vi "commit settings.vi"(8 "error in (no error)":errorcluster, 11 "Builders in":refnum<class "Builder.lvclass">) -> (0 "error out":errorcluster, 2 "Destinations":T1[](array[typedef]), 3 "Builders out":refnum<class "Builder.lvclass">)   [LabVIEW 2024, in "Builder.lvclass"]
uses:
  Builder.lvclass
  Builder.lvclass/Builder.ctl
  <vilib>/AppBuilder/AB_API/common/AB_API Destination Type.ctl
  <vilib>/AppBuilder/AB_API/common/AB_API Destination Data.ctl
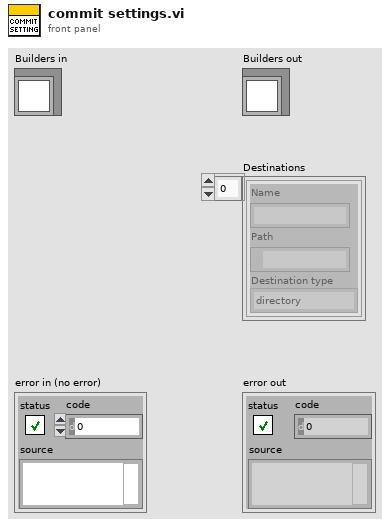
[diagram p1: front panel]
types:
  T1 = typedef "AB_API Destination Data.ctl" = cluster{"Name":string, "Path":path, "Destination type":T2}
  T2 = typedef "AB_API Destination Type.ctl" = enum16{"directory", "directory (preserve hierarchy)", "LLB"}
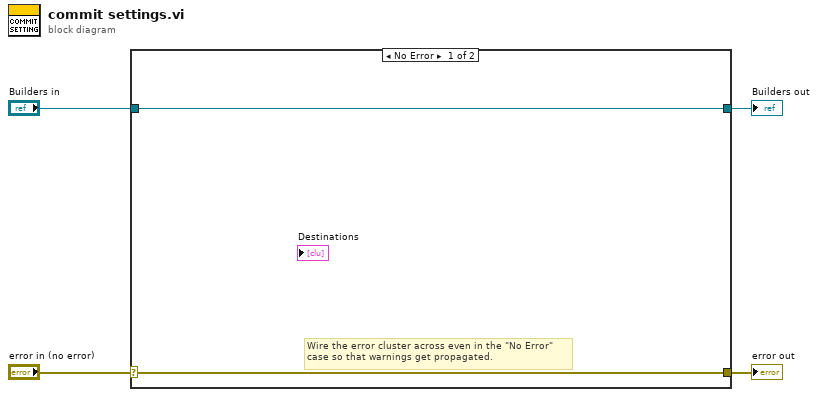
[diagram p0: block diagram]
diagram:
  n1 = case shown="No Error" "error in (no error)" {
    selector: "error in (no error)" -> [w5 w8]
    tunnel: [w5 w8] -> w3
    tunnel: [w6 w7] -> w1
    tunnel: "Builders in" -> [w6 w7]
    frame No Error {
      # "Wire the error cluster across even in the \"No Error\"\ncase so that warnings get propagated."
    }
    frame Error {
    }
  }
  "error out" <- w3
  "Builders out" <- w1
